vi "Flatten Value.vi"(8 "Error In":errorcluster, 11 "Tree Data In":refnum<class "Tree Data.lvclass">) -> (0 "Error Out":errorcluster, 1 "Value":string, 3 "Tree Data Out":refnum<class "Tree Data.lvclass">)   [LabVIEW 2017, in "Tree API.lvlib" / "Tree Data.lvclass"]
doc: "Dynamic dispatch interface for flattening Tree Data classes to string."
uses:
  Tree Data.lvclass
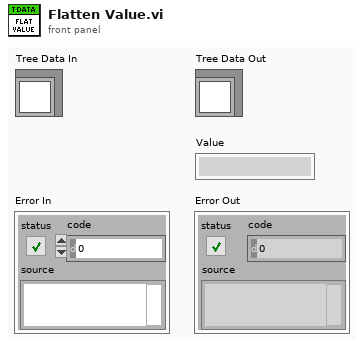
[diagram p1: front panel]
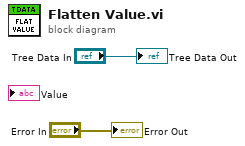
[diagram p0: block diagram]
diagram:
  "Tree Data Out" <- "Tree Data In"
  "Error Out" <- "Error In"
